vi "Shoot.vi"(11 "Button 1":bool) -> ()   [LabVIEW 2013]
uses:
  <vilib>/Rock Robotics/WPI/Solenoid/Deprecated/WPI_SolenoidSetBool.vi
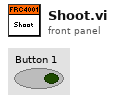
[diagram p1: front panel]
types:
  T1 = enum16{"Release Lock", "Pullback On", "Lock On", "Pullback Off"}
  T2 = typedef "WPI_SolenoidDevRef.ctl" = cluster{"DevStatus":errorcluster, "Solenoid Module":T3, "Forward Solenoid Channel":T4, "Reverse Solenoid Channel":T4}
  T3 = typedef "FPGA_TypedefSolenoidModule.ctl" = enum16{"Solenoid Module 1", "Solenoid Module 2"}
  T4 = typedef "WPI_SolenoidChannel.ctl" = enum8{"Solenoid 1", "Solenoid 2", "Solenoid 3", "Solenoid 4", "Solenoid 5", "Solenoid 6", "Solenoid 7", "Solenoid 8", "Invalid"}
  T5 = typedef "WPI_DigitalInputDevRef.ctl" = cluster{"DevStatus":errorcluster, "DIO Channel":T6, "Digital Module":T7}
  T6 = typedef "FPGA_DIOChannel.ctl" = enum8{"DIO 1", "DIO 2", "DIO 3", "DIO 4", "DIO 5", "DIO 6", "DIO 7", "DIO 8", "DIO 9", "DIO 10", "DIO 11", "DIO 12", "DIO 13", "DIO 14", "Invalid"}
  T7 = typedef "FPGA_TypedefDigitalModule.ctl" = enum16{"Digital Module 1", "Digital Module 2"}
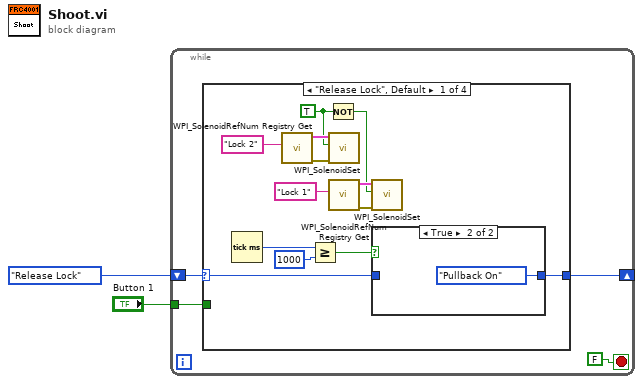
[diagram p0: block diagram]
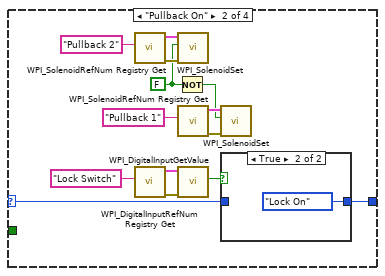
[diagram p3: hidden frame]
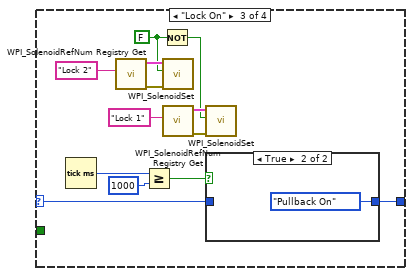
[diagram p5: hidden frame]
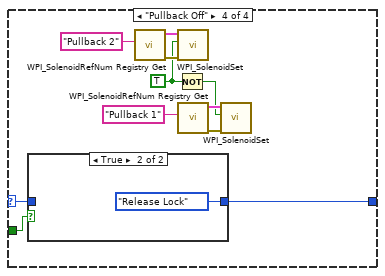
[diagram p7: hidden frame]
diagram:
  n1 = while {
    tunnel: "Button 1" -> [w5]
    shift-right: [w3] -> _
    shift-left: T1."Release Lock" -> [w4]
    stop <- FALSE stop-if-true
    n2 = case shown="\"Release Lock\", Default" w4 {
      selector: w4 -> [w11 w23 w38 w62]
      tunnel: w5 -> [_ _ _ w63]
      tunnel: [w10 w22 w39 w61] -> w3
      frame "Release Lock", Default {
        w13 = TRUE
        n3 = Tick Count (ms)() -> (millisecond timer value=w9:u32)
        n4 = call <vilib>:"WPI_SolenoidRefNum Registry Get.vi"("refnum name"="Lock 2") -> ("error out"=w14:errorcluster, "SolenoidDevRef"=w15:T2)  [unwired: 9 in]
        n5 = Greater Or Equal?(x=w9, y=u32 1000) -> (x >= y?=w7:bool)
        n6 = Not(x=w13) -> (.not. x?=w12:bool)
        n7 = call-poly <vilib>:"WPI_SolenoidSet.vi"("error in (no error)"=w14, "Value"=w13, "SolenoidDevRef"=w15) -> ()  [unwired: 7 in, 2 out]
        n8 = call <vilib>:"WPI_SolenoidRefNum Registry Get.vi"("refnum name"="Lock 1") -> ("error out"=w17:errorcluster, "SolenoidDevRef"=w18:T2)  [unwired: 9 in]
        n9 = call-poly <vilib>:"WPI_SolenoidSet.vi"("error in (no error)"=w17, "Value"=w12, "SolenoidDevRef"=w18) -> ()  [unwired: 7 in, 2 out]
        n10 = case shown="True" w7 {
          tunnel: [w20 T1."Pullback On"] -> w10
          tunnel: w11 -> [w20 _]
          frame False {
          }
          frame True {
          }
        }
      }
      frame "Pullback On" {
        w29 = FALSE
        n11 = call <vilib>:"WPI_SolenoidRefNum Registry Get.vi"("refnum name"="Pullback 2") -> ("error out"=w30:errorcluster, "SolenoidDevRef"=w31:T2)  [unwired: 9 in]
        n12 = call <vilib>:"WPI_DigitalInputRefNum Registry Get.vi"("refnum name"="Lock Switch") -> ("error out"=w27:errorcluster, "DigitalInputDevRef"=w26:T5)  [unwired: 9 in]
        n13 = Not(x=w29) -> (.not. x?=w28:bool)
        n14 = call-poly <vilib>:"WPI_SolenoidSet.vi"("error in (no error)"=w30, "Value"=w29, "SolenoidDevRef"=w31) -> ()  [unwired: 7 in, 2 out]
        n15 = call <vilib>:"WPI_SolenoidRefNum Registry Get.vi"("refnum name"="Pullback 1") -> ("error out"=w33:errorcluster, "SolenoidDevRef"=w34:T2)  [unwired: 9 in]
        n16 = call <vilib>:"WPI_DigitalInputGetValue.vi"("error in (no error)"=w27, "DigitalInputDevRef"=w26) -> ("Value"=w24:bool)  [unwired: 7 in, 2 out]
        n17 = call-poly <vilib>:"WPI_SolenoidSet.vi"("error in (no error)"=w33, "Value"=w28, "SolenoidDevRef"=w34) -> ()  [unwired: 7 in, 2 out]
        n18 = case shown="True" w24 {
          tunnel: [w36 T1."Lock On"] -> w22
          tunnel: w23 -> [w36 _]
          frame False {
          }
          frame True {
          }
        }
      }
      frame "Lock On" {
        w44 = FALSE
        n19 = Tick Count (ms)() -> (millisecond timer value=w42:u32)
        n20 = call <vilib>:"WPI_SolenoidRefNum Registry Get.vi"("refnum name"="Lock 2") -> ("error out"=w45:errorcluster, "SolenoidDevRef"=w46:T2)  [unwired: 9 in]
        n21 = Greater Or Equal?(x=w42, y=u32 1000) -> (x >= y?=w40:bool)
        n22 = Not(x=w44) -> (.not. x?=w43:bool)
        n23 = call-poly <vilib>:"WPI_SolenoidSet.vi"("error in (no error)"=w45, "Value"=w44, "SolenoidDevRef"=w46) -> ()  [unwired: 7 in, 2 out]
        n24 = call <vilib>:"WPI_SolenoidRefNum Registry Get.vi"("refnum name"="Lock 1") -> ("error out"=w48:errorcluster, "SolenoidDevRef"=w49:T2)  [unwired: 9 in]
        n25 = call-poly <vilib>:"WPI_SolenoidSet.vi"("error in (no error)"=w48, "Value"=w43, "SolenoidDevRef"=w49) -> ()  [unwired: 7 in, 2 out]
        n26 = case shown="True" w40 {
          tunnel: [w51 T1."Pullback On"] -> w39
          tunnel: w38 -> [w51 _]
          frame False {
          }
          frame True {
          }
        }
      }
      frame "Pullback Off" {
        w54 = TRUE
        n27 = case shown="True" w63 {
          tunnel: w62 -> [w64 _]
          tunnel: [w64 T1."Release Lock"] -> w61
          frame False {
          }
          frame True {
          }
        }
        n28 = call <vilib>:"WPI_SolenoidRefNum Registry Get.vi"("refnum name"="Pullback 2") -> ("error out"=w55:errorcluster, "SolenoidDevRef"=w56:T2)  [unwired: 9 in]
        n29 = Not(x=w54) -> (.not. x?=w53:bool)
        n30 = call-poly <vilib>:"WPI_SolenoidSet.vi"("error in (no error)"=w55, "Value"=w54, "SolenoidDevRef"=w56) -> ()  [unwired: 7 in, 2 out]
        n31 = call <vilib>:"WPI_SolenoidRefNum Registry Get.vi"("refnum name"="Pullback 1") -> ("error out"=w58:errorcluster, "SolenoidDevRef"=w59:T2)  [unwired: 9 in]
        n32 = call-poly <vilib>:"WPI_SolenoidSet.vi"("error in (no error)"=w58, "Value"=w53, "SolenoidDevRef"=w59) -> ()  [unwired: 7 in, 2 out]
      }
    }
  }
